vi "VFPOverloads.vi"(8 "error in (no error)":errorcluster, 11 "Overload IN":u32 format="%04x") -> (0 "error out":errorcluster, 3 "Overloads":T1)   [LabVIEW 2016]
uses:
  ol_defs.ctl
panel:
  out "Binary":u32 format="%016b"
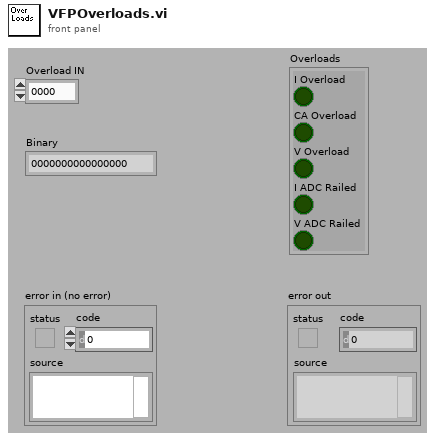
[diagram p1: front panel]
types:
  T1 = cluster{"I Overload":bool, "CA Overload":bool, "V Overload":bool, "I ADC Railed":bool, "V ADC Railed":bool}
  T2 = typedef "ol_defs.ctl" = u32
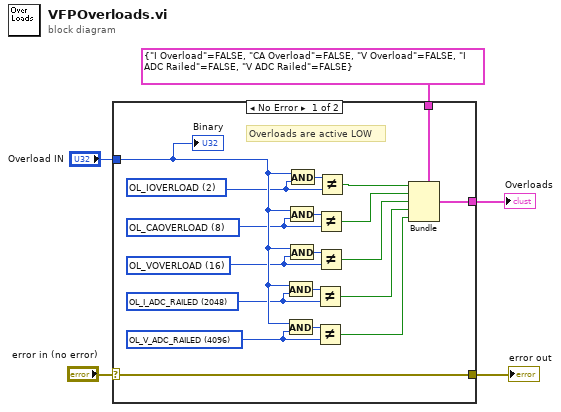
[diagram p0: block diagram]
diagram:
  n1 = case shown="No Error" "error in (no error)" {
    selector: "error in (no error)" -> [w12 w25]
    tunnel: "Overload IN" -> [w11 _]
    tunnel: T1 {"I Overload"=FALSE, "CA Overload"=FALSE, "V Overload"=FALSE, "I ADC Railed"=FALSE, "V ADC Railed"=FALSE} -> [w14 w26]
    tunnel: [w13 w26] -> w1
    tunnel: [w12 w25] -> w2
    frame No Error {
      w9 = T2 4096 items=["OL_IHISTORY"=1, "OL_IOVERLOAD"=2, "OL_CAHISTORY"=4, "OL_CAOVERLOAD"=8, "OL_VOVERLOAD"=16, "OL_OVERRUN"=32, "OL_HEATSINK_OT"=64, "OL_PWRSUPPLY_OT"=128, "OL_BOOSTER_OT"=256, "OL_H_SETTLING"=512, "OL_S_SETTLING"=1024, "OL_I_ADC_RAILED"=2048, "OL_V_ADC_RAILED"=4096, "OL_A_ADC_RAILED"=8192] ("Ring")
      w8 = T2 2048 items=["OL_IHISTORY"=1, "OL_IOVERLOAD"=2, "OL_CAHISTORY"=4, "OL_CAOVERLOAD"=8, "OL_VOVERLOAD"=16, "OL_OVERRUN"=32, "OL_HEATSINK_OT"=64, "OL_PWRSUPPLY_OT"=128, "OL_BOOSTER_OT"=256, "OL_H_SETTLING"=512, "OL_S_SETTLING"=1024, "OL_I_ADC_RAILED"=2048, "OL_V_ADC_RAILED"=4096, "OL_A_ADC_RAILED"=8192] ("Ring")
      w7 = T2 16 items=["OL_IHISTORY"=1, "OL_IOVERLOAD"=2, "OL_CAHISTORY"=4, "OL_CAOVERLOAD"=8, "OL_VOVERLOAD"=16, "OL_OVERRUN"=32, "OL_HEATSINK_OT"=64, "OL_PWRSUPPLY_OT"=128, "OL_BOOSTER_OT"=256, "OL_H_SETTLING"=512, "OL_S_SETTLING"=1024, "OL_I_ADC_RAILED"=2048, "OL_V_ADC_RAILED"=4096, "OL_A_ADC_RAILED"=8192] ("Ring")
      w6 = T2 8 items=["OL_IHISTORY"=1, "OL_IOVERLOAD"=2, "OL_CAHISTORY"=4, "OL_CAOVERLOAD"=8, "OL_VOVERLOAD"=16, "OL_OVERRUN"=32, "OL_HEATSINK_OT"=64, "OL_PWRSUPPLY_OT"=128, "OL_BOOSTER_OT"=256, "OL_H_SETTLING"=512, "OL_S_SETTLING"=1024, "OL_I_ADC_RAILED"=2048, "OL_V_ADC_RAILED"=4096, "OL_A_ADC_RAILED"=8192] ("Ring")
      w10 = T2 2 items=["OL_IHISTORY"=1, "OL_IOVERLOAD"=2, "OL_CAHISTORY"=4, "OL_CAOVERLOAD"=8, "OL_VOVERLOAD"=16, "OL_OVERRUN"=32, "OL_HEATSINK_OT"=64, "OL_PWRSUPPLY_OT"=128, "OL_BOOSTER_OT"=256, "OL_H_SETTLING"=512, "OL_S_SETTLING"=1024, "OL_I_ADC_RAILED"=2048, "OL_V_ADC_RAILED"=4096, "OL_A_ADC_RAILED"=8192] ("Ring")
      # "Overloads are active LOW"
      n2 = And(x=w11, y=w8) -> (x .and. y?=w21:T2)
      n3 = And(x=w11, y=w9) -> (x .and. y?=w20:T2)
      n4 = And(x=w11, y=w6) -> (x .and. y?=w23:T2)
      n5 = And(x=w11, y=w7) -> (x .and. y?=w22:T2)
      n6 = And(x=w11, y=w10) -> (x .and. y?=w24:T2)
      n7 = Not Equal?(x=w21, y=w8) -> (x != y?=w16:bool)
      n8 = Not Equal?(x=w20, y=w9) -> (x != y?=w15:bool)
      n9 = Not Equal?(x=w23, y=w6) -> (x != y?=w18:bool)
      n10 = Not Equal?(x=w22, y=w7) -> (x != y?=w17:bool)
      n11 = Not Equal?(x=w24, y=w10) -> (x != y?=w19:bool)
      n12 = Bundle(cluster=w14, "I Overload"=w19, "CA Overload"=w18, "V Overload"=w17, "I ADC Railed"=w16, "V ADC Railed"=w15) -> (w13:T1)
      "Binary" <- w11
    }
    frame Error {
    }
  }
  "error out" <- w2
  "Overloads" <- w1
